vi "Finish.vi"   [LabVIEW 2013]
doc: "This VI is called just before exiting. It is expected to close I/O refnum, save collected data, etc."
uses:
  <vilib>/Rock Robotics/WPI/Joystick/WPI_JoystickGetSetRefNum.vi
  <vilib>/Rock Robotics/WPI/Compressor/WPI_CompressorGetSetRefNum.vi
  <vilib>/Rock Robotics/WPI/RobotDrive/WPI_RobotDriveGetSetRefNum.vi
types:
  T1 = typedef "WPI_JoystickDevRef.ctl" = cluster{"Device":T2}
  T2 = typedef "WPI_JoystickDeviceEnum.ctl" = enum16{"USB 1", "USB 2", "USB 3", "USB 4", "Kinect 1", "Kinect 2"}
  T3 = typedef "WPI_SolenoidDevRef.ctl" = cluster{"DevStatus":errorcluster, "Solenoid Module":T4, "Forward Solenoid Channel":T5, "Reverse Solenoid Channel":T5}
  T4 = typedef "FPGA_TypedefSolenoidModule.ctl" = enum16{"Solenoid Module 1", "Solenoid Module 2"}
  T5 = typedef "WPI_SolenoidChannel.ctl" = enum8{"Solenoid 1", "Solenoid 2", "Solenoid 3", "Solenoid 4", "Solenoid 5", "Solenoid 6", "Solenoid 7", "Solenoid 8", "Invalid"}
  T6 = typedef "WPI_AnalogChannelDevRef.ctl" = cluster{"DevStatus":errorcluster, "Analog Module":T7, "Analog Channel":T8}
  T7 = typedef "FPGA_TypedefAnalogModule.ctl" = enum16{"Analog Module 1", "Analog Module 2"}
  T8 = typedef "FPGA_AIChannel.ctl" = enum8{"AI 1", "AI 2", "AI 3", "AI 4", "AI 5", "AI 6", "AI 7", "AI 8", "Invalid"}
  T9 = typedef "WPI_MotorControlDeviceRef.ctl" = cluster{"DeviceStatus":errorcluster, "Type":enum16{"PWM", "CAN"}, "PWM":cluster{"Digital Module":T10, "PWM Channel":T11, "DeadBand":T12}, "CAN":cluster{"Device Number":u8, "Control Mode":T13, "Semaphore":T14, "Max Vout":dbl}, "Invert":bool, "TransformRef":T15, "InvTransformRef":T15}
  T10 = typedef "FPGA_TypedefDigitalModule.ctl" = enum16{"Digital Module 1", "Digital Module 2"}
  T11 = typedef "FPGA_DIOPWMChannel.ctl" = enum8{"PWM 1", "PWM 2", "PWM 3", "PWM 4", "PWM 5", "PWM 6", "PWM 7", "PWM 8", "PWM 9", "PWM 10", "Invalid"}
  T12 = typedef "WPI_PWMDeadband.ctl" = cluster{"Name":string, "maxPositivePwm":i32, "minPositivePwm":i32, "centerPwm":i32, "maxNegativePwm":i32, "minNegativePwm":i32, "angularRange":u16}
  T13 = typedef "WPI_CANJaguar_ControlMode.ctl" = enum8{"Percent VBus", "Current", "Speed", "Position", "Voltage"}
  T14 = typedef "Semaphore RefNum" = refnum<k1>
  T15 = typedef "WPI_PWMTransform_ConPane.ctl" = refnum<vi>
  T16 = typedef "WPI_DigitalInputDevRef.ctl" = cluster{"DevStatus":errorcluster, "DIO Channel":T17, "Digital Module":T10}
  T17 = typedef "FPGA_DIOChannel.ctl" = enum8{"DIO 1", "DIO 2", "DIO 3", "DIO 4", "DIO 5", "DIO 6", "DIO 7", "DIO 8", "DIO 9", "DIO 10", "DIO 11", "DIO 12", "DIO 13", "DIO 14", "Invalid"}
  T18 = typedef "WPI_CompressorDevRef.ctl" = cluster{"DevStatus":errorcluster, "DigitalInputDevRef":T16, "RelayDevRef":T19}
  T19 = typedef "WPI_RelayDevRef.ctl" = cluster{"DevStatus":errorcluster, "Relay Channel":T20, "Digital Module":T10, "Relay Direction":T21}
  T20 = typedef "FPGA_DIORelayChannel.ctl" = enum8{"Relay 1", "Relay 2", "Relay 3", "Relay 4", "Relay 5", "Relay 6", "Relay 7", "Relay 8", "Invalid"}
  T21 = typedef "WPI_RelayDirection.ctl" = enum16{"Both directions", "Forward only", "Reverse only"}
  T22 = typedef "WPI_RobotDriveDevRef.ctl" = cluster{"DevStatus":errorcluster, "Motors[]":T9[], "Square Inputs":bool, "Max Output":dbl, "Isochronous":bool}
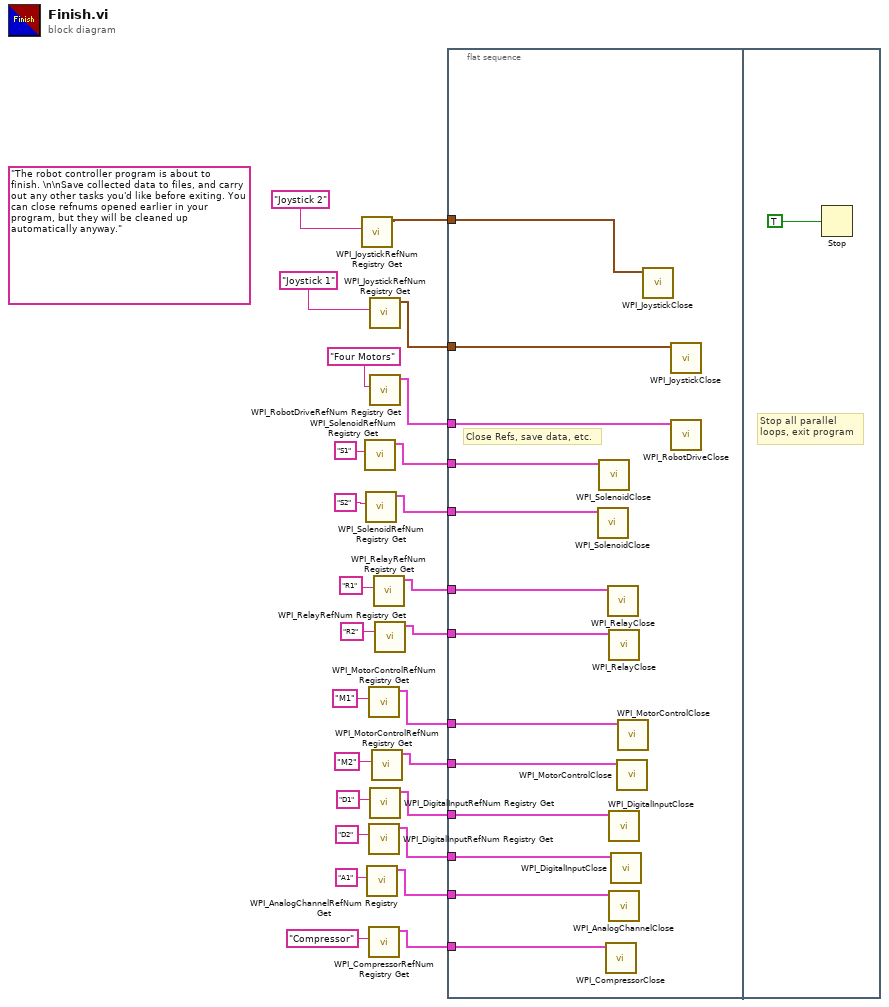
[diagram p0: block diagram]
diagram:
  (unwired) "The robot controller program is about to finish. \n\nSave collected data to files, and carry out any other tasks you'd like before exiting. You can close refnums opened earlier in your program, but they will be cleaned up automatically anyway."
  n1 = call <vilib>:"WPI_JoystickRefNum Registry Get.vi"("refnum name"="Joystick 2") -> ("JoystickDevRef"=w13:T1)  [unwired: 1 in, 9 out]
  n2 = call <vilib>:"WPI_SolenoidRefNum Registry Get.vi"("refnum name"="S1") -> ("SolenoidDevRef"=w10:T3)  [unwired: 9 in, 1 out]
  n3 = call <vilib>:"WPI_SolenoidRefNum Registry Get.vi"("refnum name"="S2") -> ("SolenoidDevRef"=w9:T3)  [unwired: 9 in, 1 out]
  n4 = call <vilib>:"WPI_AnalogChannelRefNum Registry Get.vi"("refnum name"="A1") -> ("AIDeviceRef"=w2:T6)  [unwired: 9 in, 1 out]
  n5 = call <vilib>:"WPI_MotorControlRefNum Registry Get.vi"("refnum name"="M1") -> ("MotorControlDevRef"=w6:T9)  [unwired: 9 in, 1 out]
  n6 = call <vilib>:"WPI_DigitalInputRefNum Registry Get.vi"("refnum name"="D2") -> ("DigitalInputDevRef"=w3:T16)  [unwired: 9 in, 1 out]
  n7 = call <vilib>:"WPI_CompressorRefNum Registry Get.vi"("refnum name"="Compressor") -> ("CompressorDevRef"=w1:T18)  [unwired: 9 in, 1 out]
  n8 = call <vilib>:"WPI_JoystickRefNum Registry Get.vi"("refnum name"="Joystick 1") -> ("JoystickDevRef"=w12:T1)  [unwired: 1 in, 9 out]
  n9 = call <vilib>:"WPI_RobotDriveRefNum Registry Get.vi"("refnum name"="Four Motors") -> ("RobotDriveDevRef"=w11:T22)  [unwired: 1 in, 9 out]
  n10 = call <vilib>:"WPI_DigitalInputRefNum Registry Get.vi"("refnum name"="D1") -> ("DigitalInputDevRef"=w4:T16)  [unwired: 9 in, 1 out]
  n11 = call <vilib>:"WPI_MotorControlRefNum Registry Get.vi"("refnum name"="M2") -> ("MotorControlDevRef"=w5:T9)  [unwired: 9 in, 1 out]
  n12 = call <vilib>:"WPI_RelayRefNum Registry Get.vi"("refnum name"="R1") -> ("RelayDevRef"=w8:T19)  [unwired: 9 in, 1 out]
  n13 = call <vilib>:"WPI_RelayRefNum Registry Get.vi"("refnum name"="R2") -> ("RelayDevRef"=w7:T19)  [unwired: 9 in, 1 out]
  n14 = flat-sequence {
    tunnel: w13 -> [w39]
    tunnel: w12 -> [w38]
    tunnel: w11 -> [w37]
    tunnel: w10 -> [w36]
    tunnel: w9 -> [w35]
    tunnel: w8 -> [w34]
    tunnel: w7 -> [w33]
    tunnel: w6 -> [w32]
    tunnel: w5 -> [w31]
    tunnel: w4 -> [w30]
    tunnel: w3 -> [w29]
    tunnel: w2 -> [w28]
    tunnel: w1 -> [w27]
    frame #0 {
      # "Close Refs, save data, etc."
      n15 = call <vilib>:"WPI_SolenoidClose.vi"("SolenoidDevRef"=w35) -> ()  [unwired: 10 in, 1 out]
      n16 = call <vilib>:"WPI_SolenoidClose.vi"("SolenoidDevRef"=w36) -> ()  [unwired: 10 in, 1 out]
      n17 = call <vilib>:"WPI_CompressorClose.vi"("CompressorDevRef"=w27) -> ()  [unwired: 10 in, 1 out]
      n18 = call <vilib>:"WPI_RelayClose.vi"("RelayDevRef"=w34) -> ()  [unwired: 10 in, 1 out]
      n19 = call <vilib>:"WPI_RelayClose.vi"("RelayDevRef"=w33) -> ()  [unwired: 10 in, 1 out]
      n20 = call <vilib>:"WPI_DigitalInputClose.vi"("DigitalInputDevRef"=w30) -> ()  [unwired: 10 in, 1 out]
      n21 = call <vilib>:"WPI_AnalogChannelClose.vi"("AIDeviceRef"=w28) -> ()  [unwired: 10 in, 1 out]
      n22 = call <vilib>:"WPI_DigitalInputClose.vi"("DigitalInputDevRef"=w29) -> ()  [unwired: 10 in, 1 out]
      n23 = call <vilib>:"WPI_MotorControlClose.vi"("MotorControlDevRef"=w31) -> ()  [unwired: 10 in, 1 out]
      n24 = call <vilib>:"WPI_MotorControlClose.vi"("MotorControlDevRef"=w32) -> ()  [unwired: 10 in, 1 out]
      n25 = call <vilib>:"WPI_JoystickClose.vi"("JoystickDevRef"=w39) -> ()  [unwired: 11 out]
      n26 = call <vilib>:"WPI_JoystickClose.vi"("JoystickDevRef"=w38) -> ()  [unwired: 11 out]
      n27 = call <vilib>:"WPI_RobotDriveClose.vi"("RobotDriveDevRef"=w37) -> ()  [unwired: 1 in, 10 out]
    }
    frame #1 {
      # "Stop all parallel\nloops, exit program"
      n28 = Stop(stop? (T)=TRUE ("Quit")) -> ()
    }
  }
